vi "BCU诊断标定.vi"(8 "CAN端口":u16(ring), 9 "设备索引号":u16(ring), 10 "CAN卡类型":u32(ring)=21, 11 "Myindex":dbl=1.0) -> (3 "成功":bool)   [LabVIEW 2013] (continued)
            n1896 = event-data() -> ("NewVal"=w2288:bool)  [unwired: 6 out]
            n1897 = case shown="真" w2288 {
              tunnel: w2292 -> [w2294 w2300]
              tunnel: [w2294 w2299] -> w2291
              tunnel: w2290 -> [w2293 w2298]
              tunnel: [w2293 w2297] -> w2289
              frame False {
              }
              frame True {
                n1898 = local write "布尔"(TRUE ("布尔")) -> ()
                n1899 = Enqueue Element(queue=w2300, element="读配置文件", error in (no error)=w2298) -> (queue out=w2299:refnum<queue>, error out=w2297:errorcluster)  [unwired: 2 out]
                n1900 = call <vilib>:"Set Busy.vi"() -> ()  [unwired: 4 in, 8 out]
              }
            }
          }
          event "保存主板参数": Value Change {
            n1901 = event-data() -> ("NewVal"=w2301:bool)  [unwired: 6 out]
            n1902 = case shown="真" w2301 {
              tunnel: w2305 -> [w2307 w2312]
              tunnel: [w2307 w2311] -> w2304
              tunnel: w2303 -> [w2306 w2310]
              tunnel: [w2306 w2309] -> w2302
              frame False {
              }
              frame True {
                n1903 = call <vilib>:"Set Busy.vi"() -> ()  [unwired: 4 in, 8 out]
                n1904 = Enqueue Element(queue=w2312, element="写配置文件", error in (no error)=w2310) -> (queue out=w2311:refnum<queue>, error out=w2309:errorcluster)  [unwired: 2 out]
              }
            }
          }
          event "继电器全开": Value Change {
            n1905 = event-data() -> ("NewVal"=w2313:bool)  [unwired: 6 out]
            n1906 = case shown="真" w2313 {
              tunnel: w2313 -> [_ w2316]
              frame False {
              }
              frame True {
                n1907 = stacked-sequence {
                  tunnel: w2316 -> [_ w2326 _]
                  frame #0 {
                    w2317 = FALSE ("清BUFF")
                    n1908 = local write "正级继电器"(w2317) -> ()
                    n1909 = local write "负级继电器"(w2317) -> ()
                    n1910 = local write "充电继电器"(w2317) -> ()
                    n1911 = local write "加热继电器"(w2317) -> ()
                    n1912 = local write "风机继电器"(w2317) -> ()
                    n1913 = local write "预充电继电器"(w2317) -> ()
                    n1914 = local write "继电器超时处理"(FALSE ("继电器超时处理")) -> ()
                    n1915 = local write "主从选择"(enum32{"主板", "从板"}."主板" ("主从选择")) -> ()
                    n1916 = local write "清BUFF"(FALSE ("清BUFF")) -> ()
                  }
                  frame #1 {
                    n1917 = case shown="真" w2326 {
                      selector: w2326 -> [_ w2341]
                      frame False {
                      }
                      frame True {
                        w2337 = 256.0 ("y")
                        w2328 = u32 1 ("命令序号")
                        w2327 = u8 192 ("命令")
                        n1918 = local read "动作保持时间"() -> (w2338:dbl)
                        n1919 = Quotient & Remainder(x=w2338, y=w2337) -> (x-y*floor(x/y)=w2330:dbl, floor(x/y)=w2334:dbl)
                        n1920 = Quotient & Remainder(x=w2334, y=w2337) -> (x-y*floor(x/y)=w2331:dbl, floor(x/y)=w2335:dbl)
                        n1921 = Quotient & Remainder(x=w2335, y=w2337) -> (x-y*floor(x/y)=w2332:dbl, floor(x/y)=w2336:dbl)
                        n1922 = local read "设备索引号"() -> (w2345:u16)
                        n1923 = local read "CAN卡类型"() -> (w2346:u32)
                        n1924 = local read "CAN端口"() -> (w2344:u16)
                        n1925 = Boolean To (0,1)(Boolean=w2341) -> (0, 1=w2339:i16)
                        n1926 = Quotient & Remainder(x=w2336, y=w2337) -> (x-y*floor(x/y)=w2333:dbl)  [unwired: 1 out]
                        n1927 = Build Array(i16 170 ("元素"), w2339, w2333, w2332, w2331, w2330, 0.0 ("元素")) -> (w2342:dbl[])
                        n1928 = call "多帧发送机制(EV05).vi"("can卡类型"=w2346, "设备索引号"=w2345, "CAN端口"=w2344, "命令"=w2327, "板号"=u8 0, "命令序号"=w2328, "输入数据"=w2342) -> ()  [unwired: 2 in, 11 out]
                        n1929 = local write "命令序号"(w2328) -> ()
                        n1930 = local write "命令"(w2327) -> ()
                      }
                    }
                    n1931 = local write "控制1"(TRUE ("控制1")) -> ()
                    n1932 = local write "写?"(FALSE ("写?")) -> ()
                    n1933 = local write "消除"(TRUE ("消除")) -> ()
                    n1934 = global write "EV05全局变量1.vi" "流控帧 2"(TRUE ("流控帧 2")) -> ()
                    n1935 = global write "EV05全局变量1.vi" "流控帧"(FALSE ("流控帧")) -> ()
                  }
                  frame #2 {
                    n1936 = flat-sequence {
                      tunnel: [w2348] -> w2347
                      tunnel: w2347 -> [w2355]
                      frame #0 {
                        n1937 = while {
                          tunnel: [w2349] -> w2348
                          i -> [w2353]
                          stop <- w2350 stop-if-true
                          n1938 = local read "继电器超时处理"() -> (w2349:bool)
                          n1939 = Greater Or Equal?(x=w2353, y=20) -> (x >= y?=w2351:bool)
                          n1940 = Wait Until Next ms Multiple(millisecond multiple=u32 100 ("毫秒倍数")) -> ()  [unwired: 1 out]
                          n1941 = Or(x=w2349, y=w2351) -> (x .or. y?=w2350:bool)
                        }
                      }
                      frame #1 {
                        n1942 = case shown="真" w2355 {
                          frame False {
                            n1943 = One Button Dialog(message="继电器处理超时" ("消息"), button name ("OK")="是" ("按钮名称（“确定”）")) -> ()  [unwired: 1 out]
                          }
                          frame True {
                            w2358 = TRUE ("清BUFF")
                            n1944 = local write "正级继电器"(w2358) -> ()
                            n1945 = local write "负级继电器"(w2358) -> ()
                            n1946 = local write "充电继电器"(w2358) -> ()
                            n1947 = local write "加热继电器"(w2358) -> ()
                            n1948 = local write "风机继电器"(w2358) -> ()
                            n1949 = local write "预充电继电器"(w2358) -> ()
                          }
                        }
                      }
                    }
                  }
                }
              }
            }
          }
          event "继电器全关": Value Change {
            n1950 = event-data() -> ("NewVal"=w2359:bool)  [unwired: 6 out]
            n1951 = case shown="真" w2359 {
              tunnel: w2359 -> [_ w2362]
              frame False {
              }
              frame True {
                n1952 = stacked-sequence {
                  tunnel: w2362 -> [_ w2372 _]
                  frame #0 {
                    w2363 = TRUE ("清BUFF")
                    n1953 = local write "正级继电器"(w2363) -> ()
                    n1954 = local write "负级继电器"(w2363) -> ()
                    n1955 = local write "充电继电器"(w2363) -> ()
                    n1956 = local write "加热继电器"(w2363) -> ()
                    n1957 = local write "风机继电器"(w2363) -> ()
                    n1958 = local write "预充电继电器"(w2363) -> ()
                    n1959 = local write "继电器超时处理"(FALSE ("继电器超时处理")) -> ()
                    n1960 = local write "主从选择"(enum32{"主板", "从板"}."主板" ("主从选择")) -> ()
                    n1961 = global write "EV05全局变量1.vi" "流控帧"(FALSE ("流控帧")) -> ()
                    n1962 = local write "清BUFF"(FALSE ("清BUFF")) -> ()
                  }
                  frame #1 {
                    n1963 = case shown="真" w2372 {
                      selector: w2372 -> [_ w2387]
                      frame False {
                      }
                      frame True {
                        w2383 = 256.0 ("y")
                        w2374 = u32 1 ("命令序号")
                        w2373 = u8 192 ("命令")
                        n1964 = local read "动作保持时间"() -> (w2384:dbl)
                        n1965 = Quotient & Remainder(x=w2384, y=w2383) -> (x-y*floor(x/y)=w2376:dbl, floor(x/y)=w2380:dbl)
                        n1966 = Quotient & Remainder(x=w2380, y=w2383) -> (x-y*floor(x/y)=w2377:dbl, floor(x/y)=w2381:dbl)
                        n1967 = Quotient & Remainder(x=w2381, y=w2383) -> (x-y*floor(x/y)=w2378:dbl, floor(x/y)=w2382:dbl)
                        n1968 = local read "设备索引号"() -> (w2391:u16)
                        n1969 = local read "CAN卡类型"() -> (w2392:u32)
                        n1970 = local read "CAN端口"() -> (w2390:u16)
                        n1971 = Boolean To (0,1)(Boolean=w2387) -> (0, 1=w2385:i16)
                        n1972 = Quotient & Remainder(x=w2382, y=w2383) -> (x-y*floor(x/y)=w2379:dbl)  [unwired: 1 out]
                        n1973 = Build Array(i16 85 ("元素"), w2385, w2379, w2378, w2377, w2376, 0.0 ("元素")) -> (w2388:dbl[])
                        n1974 = call "多帧发送机制(EV05).vi"("can卡类型"=w2392, "设备索引号"=w2391, "CAN端口"=w2390, "命令"=w2373, "板号"=u8 0, "命令序号"=w2374, "输入数据"=w2388) -> ()  [unwired: 2 in, 11 out]
                        n1975 = local write "命令序号"(w2374) -> ()
                        n1976 = local write "命令"(w2373) -> ()
                      }
                    }
                    n1977 = local write "控制1"(TRUE ("控制1")) -> ()
                    n1978 = local write "写?"(FALSE ("写?")) -> ()
                    n1979 = local write "消除"(TRUE ("消除")) -> ()
                    n1980 = global write "EV05全局变量1.vi" "流控帧 2"(TRUE ("流控帧 2")) -> ()
                  }
                  frame #2 {
                    n1981 = flat-sequence {
                      tunnel: [w2394] -> w2393
                      tunnel: w2393 -> [w2401]
                      frame #0 {
                        n1982 = while {
                          tunnel: [w2395] -> w2394
                          i -> [w2399]
                          stop <- w2396 stop-if-true
                          n1983 = local read "继电器超时处理"() -> (w2395:bool)
                          n1984 = Greater Or Equal?(x=w2399, y=20) -> (x >= y?=w2397:bool)
                          n1985 = Wait Until Next ms Multiple(millisecond multiple=u32 100 ("毫秒倍数")) -> ()  [unwired: 1 out]
                          n1986 = Or(x=w2395, y=w2397) -> (x .or. y?=w2396:bool)
                        }
                      }
                      frame #1 {
                        n1987 = case shown="真" w2401 {
                          frame False {
                            n1988 = One Button Dialog(message="继电器处理超时" ("消息"), button name ("OK")="是" ("按钮名称（“确定”）")) -> ()  [unwired: 1 out]
                          }
                          frame True {
                            w2404 = FALSE ("清BUFF")
                            n1989 = local write "正级继电器"(w2404) -> ()
                            n1990 = local write "负级继电器"(w2404) -> ()
                            n1991 = local write "充电继电器"(w2404) -> ()
                            n1992 = local write "加热继电器"(w2404) -> ()
                            n1993 = local write "风机继电器"(w2404) -> ()
                            n1994 = local write "预充电继电器"(w2404) -> ()
                          }
                        }
                      }
                    }
                  }
                }
              }
            }
          }
          event "控制按键全为开": Value Change {
            n1995 = event-data() -> ("NewVal"=w2405:bool)  [unwired: 6 out]
            n1996 = case shown="真" w2405 {
              frame False {
              }
              frame True {
                w2406 = TRUE ("正级继电器")
                n1997 = local write "加热继电器(从)"(w2406) -> ()
                n1998 = local write "风机继电器(从)"(w2406) -> ()
                n1999 = local write "DO1 2"(w2406) -> ()
                n2000 = local write "DO1"(w2406) -> ()
                n2001 = local write "DO2"(w2406) -> ()
                n2002 = local write "正级继电器"(w2406) -> ()
                n2003 = local write "负级继电器"(w2406) -> ()
                n2004 = local write "加热继电器"(w2406) -> ()
                n2005 = local write "预充电继电器"(w2406) -> ()
                n2006 = local write "充电继电器"(w2406) -> ()
                n2007 = local write "风机继电器"(w2406) -> ()
              }
            }
          }
          event "控制按键全为关": Value Change {
            n2008 = event-data() -> ("NewVal"=w2407:bool)  [unwired: 6 out]
            n2009 = case shown="真" w2407 {
              frame False {
              }
              frame True {
                w2408 = FALSE ("正级继电器")
                n2010 = local write "加热继电器(从)"(w2408) -> ()
                n2011 = local write "风机继电器(从)"(w2408) -> ()
                n2012 = local write "DO1 2"(w2408) -> ()
                n2013 = local write "DO1"(w2408) -> ()
                n2014 = local write "DO2"(w2408) -> ()
                n2015 = local write "正级继电器"(w2408) -> ()
                n2016 = local write "负级继电器"(w2408) -> ()
                n2017 = local write "加热继电器"(w2408) -> ()
                n2018 = local write "预充电继电器"(w2408) -> ()
                n2019 = local write "充电继电器"(w2408) -> ()
                n2020 = local write "风机继电器"(w2408) -> ()
              }
            }
          }
          event "正级继电器": Value Change {
            n2021 = event-data() -> ("NewVal"=w2409:bool)  [unwired: 6 out]
            n2022 = stacked-sequence {
              tunnel: w2409 -> [_ w2422 _]
              frame #0 {
                w2412 = FALSE ("清BUFF")
                n2023 = local write "继电器超时处理"(FALSE ("继电器超时处理")) -> ()
                n2024 = local write "主从选择"(enum32{"主板", "从板"}."主板" ("主从选择")) -> ()
                n2025 = local write "正级继电器 12"(w2412) -> ()
                n2026 = local write "清BUFF"(w2412) -> ()
              }
              frame #1 {
                n2027 = case shown="假" w2422 {
                  selector: w2422 -> [w2437 w2457]
                  tunnel: [w2436 w2456] -> w2421
                  tunnel: [w2424 w2444] -> w2416
                  frame False {
                    w2432 = 256.0 ("y")
                    w2424 = u32 1 ("命令序号")
                    w2436 = u8 192 ("命令")
                    n2028 = local read "动作保持时间"() -> (w2433:dbl)
                    n2029 = Quotient & Remainder(x=w2433, y=w2432) -> (x-y*floor(x/y)=w2425:dbl, floor(x/y)=w2429:dbl)
                    n2030 = Quotient & Remainder(x=w2429, y=w2432) -> (x-y*floor(x/y)=w2426:dbl, floor(x/y)=w2430:dbl)
                    n2031 = Quotient & Remainder(x=w2430, y=w2432) -> (x-y*floor(x/y)=w2427:dbl, floor(x/y)=w2431:dbl)
                    n2032 = local read "设备索引号"() -> (w2441:u16)
                    n2033 = local read "CAN卡类型"() -> (w2442:u32)
                    n2034 = local read "CAN端口"() -> (w2440:u16)
                    n2035 = Boolean To (0,1)(Boolean=w2437) -> (0, 1=w2434:i16)
                    n2036 = Quotient & Remainder(x=w2431, y=w2432) -> (x-y*floor(x/y)=w2428:dbl)  [unwired: 1 out]
                    n2037 = Build Array(i16 1 ("元素"), w2434, w2428, w2427, w2426, w2425, 0.0 ("元素")) -> (w2438:dbl[])
                    n2038 = call "多帧发送机制(EV05).vi"("can卡类型"=w2442, "设备索引号"=w2441, "CAN端口"=w2440, "命令"=w2436, "板号"=u8 0, "命令序号"=w2424, "输入数据"=w2438) -> ()  [unwired: 2 in, 11 out]
                  }
                  frame True {
                    w2452 = 256.0 ("y")
                    w2444 = u32 1 ("命令序号")
                    w2456 = u8 192 ("命令")
                    n2039 = local read "动作保持时间"() -> (w2453:dbl)
                    n2040 = Quotient & Remainder(x=w2453, y=w2452) -> (x-y*floor(x/y)=w2445:dbl, floor(x/y)=w2449:dbl)
                    n2041 = Quotient & Remainder(x=w2449, y=w2452) -> (x-y*floor(x/y)=w2446:dbl, floor(x/y)=w2450:dbl)
                    n2042 = Quotient & Remainder(x=w2450, y=w2452) -> (x-y*floor(x/y)=w2447:dbl, floor(x/y)=w2451:dbl)
                    n2043 = local read "设备索引号"() -> (w2461:u16)
                    n2044 = local read "CAN卡类型"() -> (w2462:u32)
                    n2045 = local read "CAN端口"() -> (w2460:u16)
                    n2046 = Boolean To (0,1)(Boolean=w2457) -> (0, 1=w2454:i16)
                    n2047 = Quotient & Remainder(x=w2451, y=w2452) -> (x-y*floor(x/y)=w2448:dbl)  [unwired: 1 out]
                    n2048 = Build Array(i16 1 ("元素"), w2454, w2448, w2447, w2446, w2445, 0.0 ("元素")) -> (w2458:dbl[])
                    n2049 = call "多帧发送机制(EV05).vi"("can卡类型"=w2462, "设备索引号"=w2461, "CAN端口"=w2460, "命令"=w2456, "板号"=u8 0, "命令序号"=w2444, "输入数据"=w2458) -> ()  [unwired: 2 in, 11 out]
                  }
                }
                n2050 = local write "命令序号"(w2416) -> ()
                n2051 = local write "命令"(w2421) -> ()
                n2052 = local write "控制1"(TRUE ("控制1")) -> ()
                n2053 = local write "写?"(FALSE ("写?")) -> ()
                n2054 = global write "EV05全局变量1.vi" "流控帧"(FALSE ("流控帧")) -> ()
                n2055 = local write "消除"(TRUE ("消除")) -> ()
                n2056 = global write "EV05全局变量1.vi" "流控帧 2"(TRUE ("流控帧 2")) -> ()
              }
              frame #2 {
                n2057 = flat-sequence {
                  tunnel: [w2464] -> w2463
                  tunnel: w2463 -> [w2471]
                  frame #0 {
                    n2058 = while {
                      tunnel: [w2465] -> w2464
                      i -> [w2469]
                      stop <- w2466 stop-if-true
                      n2059 = local read "继电器超时处理"() -> (w2465:bool)
                      n2060 = Greater Or Equal?(x=w2469, y=20) -> (x >= y?=w2467:bool)
                      n2061 = Wait Until Next ms Multiple(millisecond multiple=u32 100 ("毫秒倍数")) -> ()  [unwired: 1 out]
                      n2062 = Or(x=w2465, y=w2467) -> (x .or. y?=w2466:bool)
                    }
                  }
                  frame #1 {
                    n2063 = case shown="假" w2471 {
                      frame False {
                        n2064 = local read "正级继电器"() -> (w2473:bool)
                        n2065 = Not(x=w2473) -> (.not. x?=w2472:bool)
                        n2066 = local write "正级继电器"(w2472) -> ()
                        n2067 = One Button Dialog(message="继电器处理超时" ("消息"), button name ("OK")="是" ("按钮名称（“确定”）")) -> ()  [unwired: 1 out]
                      }
                      frame True {
                      }
                    }
                  }
                }
              }
            }
          }
          event "负级继电器": Value Change {
            n2068 = event-data() -> ("NewVal"=w2476:bool)  [unwired: 6 out]
            n2069 = stacked-sequence {
              tunnel: w2476 -> [_ w2489 _]
              frame #0 {
                w2479 = FALSE ("继电器超时处理")
                n2070 = local write "继电器超时处理"(w2479) -> ()
                n2071 = local write "正级继电器 2"(w2479) -> ()
                n2072 = local write "主从选择"(enum32{"主板", "从板"}."主板" ("主从选择")) -> ()
              }
              frame #1 {
                n2073 = case shown="假" w2489 {
                  selector: w2489 -> [w2503 w2523]
                  tunnel: [w2502 w2522] -> w2488
                  tunnel: [w2491 w2511] -> w2483
                  frame False {
                    w2499 = 256.0 ("y")
                    w2491 = u32 1 ("命令序号")
                    w2502 = u8 192 ("命令")
                    n2074 = local read "动作保持时间"() -> (w2500:dbl)
                    n2075 = Quotient & Remainder(x=w2500, y=w2499) -> (x-y*floor(x/y)=w2492:dbl, floor(x/y)=w2496:dbl)
                    n2076 = Quotient & Remainder(x=w2496, y=w2499) -> (x-y*floor(x/y)=w2493:dbl, floor(x/y)=w2497:dbl)
                    n2077 = Quotient & Remainder(x=w2497, y=w2499) -> (x-y*floor(x/y)=w2494:dbl, floor(x/y)=w2498:dbl)
                    n2078 = Quotient & Remainder(x=w2498, y=w2499) -> (x-y*floor(x/y)=w2495:dbl)  [unwired: 1 out]
                    n2079 = Boolean To (0,1)(Boolean=w2503) -> (0, 1=w2501:i16)
                    n2080 = local read "设备索引号"() -> (w2508:u16)
                    n2081 = local read "CAN卡类型"() -> (w2509:u32)
                    n2082 = local read "CAN端口"() -> (w2507:u16)
                    n2083 = Build Array(i16 2 ("元素"), w2501, w2495, w2494, w2493, w2492, 0.0 ("元素")) -> (w2505:dbl[])
                    n2084 = call "多帧发送机制(EV05).vi"("can卡类型"=w2509, "设备索引号"=w2508, "CAN端口"=w2507, "命令"=w2502, "板号"=u8 0, "命令序号"=w2491, "输入数据"=w2505) -> ()  [unwired: 2 in, 11 out]
                  }
                  frame True {
                    w2519 = 256.0 ("y")
                    w2511 = u32 1 ("命令序号")
                    w2522 = u8 192 ("命令")
                    n2085 = local read "动作保持时间"() -> (w2520:dbl)
                    n2086 = Quotient & Remainder(x=w2520, y=w2519) -> (x-y*floor(x/y)=w2512:dbl, floor(x/y)=w2516:dbl)
                    n2087 = Quotient & Remainder(x=w2516, y=w2519) -> (x-y*floor(x/y)=w2513:dbl, floor(x/y)=w2517:dbl)
                    n2088 = Quotient & Remainder(x=w2517, y=w2519) -> (x-y*floor(x/y)=w2514:dbl, floor(x/y)=w2518:dbl)
                    n2089 = Quotient & Remainder(x=w2518, y=w2519) -> (x-y*floor(x/y)=w2515:dbl)  [unwired: 1 out]
                    n2090 = Boolean To (0,1)(Boolean=w2523) -> (0, 1=w2521:i16)
                    n2091 = local read "设备索引号"() -> (w2528:u16)
                    n2092 = local read "CAN卡类型"() -> (w2529:u32)
                    n2093 = local read "CAN端口"() -> (w2527:u16)
                    n2094 = Build Array(i16 2 ("元素"), w2521, w2515, w2514, w2513, w2512, 0.0 ("元素")) -> (w2525:dbl[])
                    n2095 = call "多帧发送机制(EV05).vi"("can卡类型"=w2529, "设备索引号"=w2528, "CAN端口"=w2527, "命令"=w2522, "板号"=u8 0, "命令序号"=w2511, "输入数据"=w2525) -> ()  [unwired: 2 in, 11 out]
                  }
                }
                n2096 = local write "命令"(w2488) -> ()
                n2097 = local write "命令序号"(w2483) -> ()
                n2098 = local write "清BUFF"(FALSE ("清BUFF")) -> ()
                n2099 = global write "EV05全局变量1.vi" "流控帧"(FALSE ("流控帧")) -> ()
                n2100 = local write "控制1"(TRUE ("控制1")) -> ()
                n2101 = global write "EV05全局变量1.vi" "流控帧 2"(TRUE ("流控帧 2")) -> ()
                n2102 = local write "写?"(FALSE ("写?")) -> ()
                n2103 = local write "消除"(TRUE ("消除")) -> ()
              }
              frame #2 {
                n2104 = flat-sequence {
                  tunnel: [w2531] -> w2530
                  tunnel: w2530 -> [w2538]
                  frame #0 {
                    n2105 = while {
                      tunnel: [w2532] -> w2531
                      i -> [w2536]
                      stop <- w2533 stop-if-true
                      n2106 = local read "继电器超时处理"() -> (w2532:bool)
                      n2107 = Greater Or Equal?(x=w2536, y=20) -> (x >= y?=w2534:bool)
                      n2108 = Wait Until Next ms Multiple(millisecond multiple=u32 100 ("毫秒倍数")) -> ()  [unwired: 1 out]
                      n2109 = Or(x=w2532, y=w2534) -> (x .or. y?=w2533:bool)
                    }
                  }
                  frame #1 {
                    n2110 = case shown="假" w2538 {
                      frame False {
                        n2111 = local read "负级继电器"() -> (w2539:bool)
                        n2112 = Not(x=w2539) -> (.not. x?=w2540:bool)
                        n2113 = local write "负级继电器"(w2540) -> ()
                        n2114 = One Button Dialog(message="继电器处理超时" ("消息"), button name ("OK")="是" ("按钮名称（“确定”）")) -> ()  [unwired: 1 out]
                      }
                      frame True {
                      }
                    }
                  }
                }
              }
            }
          }
          event "预充电继电器": Value Change {
            n2115 = event-data() -> ("NewVal"=w2543:bool)  [unwired: 6 out]
            n2116 = stacked-sequence {
              tunnel: w2543 -> [_ w2556 _]
              frame #0 {
                w2547 = FALSE ("继电器超时处理")
                n2117 = local write "继电器超时处理"(w2547) -> ()
                n2118 = local write "正级继电器 3"(w2547) -> ()
                n2119 = global write "EV05全局变量1.vi" "流控帧"(FALSE ("流控帧")) -> ()
                n2120 = local write "主从选择"(enum32{"主板", "从板"}."主板" ("主从选择")) -> ()
              }
              frame #1 {
                n2121 = case shown="假" w2556 {
                  selector: w2556 -> [w2570 w2590]
                  tunnel: [w2569 w2589] -> w2555
                  tunnel: [w2558 w2578] -> w2550
                  frame False {
                    w2566 = 256.0 ("y")
                    w2558 = u32 1 ("命令序号")
                    w2569 = u8 192 ("命令")
                    n2122 = local read "动作保持时间"() -> (w2567:dbl)
                    n2123 = Quotient & Remainder(x=w2567, y=w2566) -> (x-y*floor(x/y)=w2559:dbl, floor(x/y)=w2563:dbl)
                    n2124 = Quotient & Remainder(x=w2563, y=w2566) -> (x-y*floor(x/y)=w2560:dbl, floor(x/y)=w2564:dbl)
                    n2125 = Quotient & Remainder(x=w2564, y=w2566) -> (x-y*floor(x/y)=w2561:dbl, floor(x/y)=w2565:dbl)
                    n2126 = Quotient & Remainder(x=w2565, y=w2566) -> (x-y*floor(x/y)=w2562:dbl)  [unwired: 1 out]
                    n2127 = Boolean To (0,1)(Boolean=w2570) -> (0, 1=w2568:i16)
                    n2128 = local read "设备索引号"() -> (w2575:u16)
                    n2129 = local read "CAN卡类型"() -> (w2576:u32)
                    n2130 = local read "CAN端口"() -> (w2574:u16)
                    n2131 = Build Array(i16 3 ("元素"), w2568, w2562, w2561, w2560, w2559, 0.0 ("元素")) -> (w2572:dbl[])
                    n2132 = call "多帧发送机制(EV05).vi"("can卡类型"=w2576, "设备索引号"=w2575, "CAN端口"=w2574, "命令"=w2569, "板号"=u8 0, "命令序号"=w2558, "输入数据"=w2572) -> ()  [unwired: 2 in, 11 out]
                  }
                  frame True {
                    w2586 = 256.0 ("y")
                    w2578 = u32 1 ("命令序号")
                    w2589 = u8 192 ("命令")
                    n2133 = local read "动作保持时间"() -> (w2587:dbl)
                    n2134 = Quotient & Remainder(x=w2587, y=w2586) -> (x-y*floor(x/y)=w2579:dbl, floor(x/y)=w2583:dbl)
                    n2135 = Quotient & Remainder(x=w2583, y=w2586) -> (x-y*floor(x/y)=w2580:dbl, floor(x/y)=w2584:dbl)
                    n2136 = Quotient & Remainder(x=w2584, y=w2586) -> (x-y*floor(x/y)=w2581:dbl, floor(x/y)=w2585:dbl)
                    n2137 = Quotient & Remainder(x=w2585, y=w2586) -> (x-y*floor(x/y)=w2582:dbl)  [unwired: 1 out]
                    n2138 = Boolean To (0,1)(Boolean=w2590) -> (0, 1=w2588:i16)
                    n2139 = local read "设备索引号"() -> (w2595:u16)
                    n2140 = local read "CAN卡类型"() -> (w2596:u32)
                    n2141 = local read "CAN端口"() -> (w2594:u16)
                    n2142 = Build Array(i16 3 ("元素"), w2588, w2582, w2581, w2580, w2579, 0.0 ("元素")) -> (w2592:dbl[])
                    n2143 = call "多帧发送机制(EV05).vi"("can卡类型"=w2596, "设备索引号"=w2595, "CAN端口"=w2594, "命令"=w2589, "板号"=u8 0, "命令序号"=w2578, "输入数据"=w2592) -> ()  [unwired: 2 in, 11 out]
                  }
                }
                n2144 = local write "命令序号"(w2550) -> ()
                n2145 = local write "清BUFF"(FALSE ("清BUFF")) -> ()
                n2146 = local write "控制1"(TRUE ("控制1")) -> ()
                n2147 = global write "EV05全局变量1.vi" "流控帧 2"(TRUE ("流控帧 2")) -> ()
                n2148 = local write "消除"(TRUE ("消除")) -> ()
                n2149 = local write "命令"(w2555) -> ()
                n2150 = local write "写?"(FALSE ("写?")) -> ()
              }
              frame #2 {
                n2151 = flat-sequence {
                  tunnel: [w2598] -> w2597
                  tunnel: w2597 -> [w2605]
                  frame #0 {
                    n2152 = while {
                      tunnel: [w2599] -> w2598
                      i -> [w2603]
                      stop <- w2600 stop-if-true
                      n2153 = local read "继电器超时处理"() -> (w2599:bool)
                      n2154 = Greater Or Equal?(x=w2603, y=20) -> (x >= y?=w2601:bool)
                      n2155 = Wait Until Next ms Multiple(millisecond multiple=u32 100 ("毫秒倍数")) -> ()  [unwired: 1 out]
                      n2156 = Or(x=w2599, y=w2601) -> (x .or. y?=w2600:bool)
                    }
                  }
                  frame #1 {
                    n2157 = case shown="假" w2605 {
                      frame False {
                        n2158 = local read "预充电继电器"() -> (w2606:bool)
                        n2159 = Not(x=w2606) -> (.not. x?=w2607:bool)
                        n2160 = local write "预充电继电器"(w2607) -> ()
                        n2161 = One Button Dialog(message="继电器处理超时" ("消息"), button name ("OK")="是" ("按钮名称（“确定”）")) -> ()  [unwired: 1 out]
                      }
                      frame True {
                      }
                    }
                  }
                }
              }
            }
          }
          event "加热继电器": Value Change {
            n2162 = event-data() -> ("NewVal"=w2610:bool)  [unwired: 6 out]
            n2163 = stacked-sequence {
              tunnel: w2610 -> [_ w2623 _]
              frame #0 {
                w2614 = FALSE ("继电器超时处理")
                n2164 = local write "继电器超时处理"(w2614) -> ()
                n2165 = local write "正级继电器 5"(w2614) -> ()
                n2166 = global write "EV05全局变量1.vi" "流控帧"(FALSE ("流控帧")) -> ()
                n2167 = local write "主从选择"(enum32{"主板", "从板"}."主板" ("主从选择")) -> ()
              }
              frame #1 {
                n2168 = case shown="假" w2623 {
                  selector: w2623 -> [w2637 w2657]
                  tunnel: [w2636 w2656] -> w2622
                  tunnel: [w2625 w2645] -> w2617
                  frame False {
                    w2633 = 256.0 ("y")
                    w2625 = u32 1 ("命令序号")
                    w2636 = u8 192 ("命令")
                    n2169 = local read "动作保持时间"() -> (w2634:dbl)
                    n2170 = Quotient & Remainder(x=w2634, y=w2633) -> (x-y*floor(x/y)=w2626:dbl, floor(x/y)=w2630:dbl)
                    n2171 = Quotient & Remainder(x=w2630, y=w2633) -> (x-y*floor(x/y)=w2627:dbl, floor(x/y)=w2631:dbl)
                    n2172 = Quotient & Remainder(x=w2631, y=w2633) -> (x-y*floor(x/y)=w2628:dbl, floor(x/y)=w2632:dbl)
                    n2173 = Quotient & Remainder(x=w2632, y=w2633) -> (x-y*floor(x/y)=w2629:dbl)  [unwired: 1 out]
                    n2174 = Boolean To (0,1)(Boolean=w2637) -> (0, 1=w2635:i16)
                    n2175 = local read "设备索引号"() -> (w2642:u16)
                    n2176 = local read "CAN卡类型"() -> (w2643:u32)
                    n2177 = local read "CAN端口"() -> (w2641:u16)
                    n2178 = Build Array(i16 4 ("元素"), w2635, w2629, w2628, w2627, w2626, 0.0 ("元素")) -> (w2639:dbl[])
                    n2179 = call "多帧发送机制(EV05).vi"("can卡类型"=w2643, "设备索引号"=w2642, "CAN端口"=w2641, "命令"=w2636, "板号"=u8 0, "命令序号"=w2625, "输入数据"=w2639) -> ()  [unwired: 2 in, 11 out]
                  }
                  frame True {
                    w2653 = 256.0 ("y")
                    w2645 = u32 1 ("命令序号")
                    w2656 = u8 192 ("命令")
                    n2180 = local read "动作保持时间"() -> (w2654:dbl)
                    n2181 = Quotient & Remainder(x=w2654, y=w2653) -> (x-y*floor(x/y)=w2646:dbl, floor(x/y)=w2650:dbl)
                    n2182 = Quotient & Remainder(x=w2650, y=w2653) -> (x-y*floor(x/y)=w2647:dbl, floor(x/y)=w2651:dbl)
                    n2183 = Quotient & Remainder(x=w2651, y=w2653) -> (x-y*floor(x/y)=w2648:dbl, floor(x/y)=w2652:dbl)
                    n2184 = Quotient & Remainder(x=w2652, y=w2653) -> (x-y*floor(x/y)=w2649:dbl)  [unwired: 1 out]
                    n2185 = Boolean To (0,1)(Boolean=w2657) -> (0, 1=w2655:i16)
                    n2186 = local read "设备索引号"() -> (w2662:u16)
                    n2187 = local read "CAN卡类型"() -> (w2663:u32)
                    n2188 = local read "CAN端口"() -> (w2661:u16)
                    n2189 = Build Array(i16 4 ("元素"), w2655, w2649, w2648, w2647, w2646, 0.0 ("元素")) -> (w2659:dbl[])
                    n2190 = call "多帧发送机制(EV05).vi"("can卡类型"=w2663, "设备索引号"=w2662, "CAN端口"=w2661, "命令"=w2656, "板号"=u8 0, "命令序号"=w2645, "输入数据"=w2659) -> ()  [unwired: 2 in, 11 out]
                  }
                }
                n2191 = local write "命令序号"(w2617) -> ()
                n2192 = local write "清BUFF"(FALSE ("清BUFF")) -> ()
                n2193 = local write "命令"(w2622) -> ()
                n2194 = local write "控制1"(TRUE ("控制1")) -> ()
                n2195 = local write "写?"(FALSE ("写?")) -> ()
                n2196 = global write "EV05全局变量1.vi" "流控帧 2"(TRUE ("流控帧 2")) -> ()
                n2197 = local write "消除"(TRUE ("消除")) -> ()
              }
              frame #2 {
                n2198 = flat-sequence {
                  tunnel: [w2665] -> w2664
                  tunnel: w2664 -> [w2672]
                  frame #0 {
                    n2199 = while {
                      tunnel: [w2666] -> w2665
                      i -> [w2670]
                      stop <- w2667 stop-if-true
                      n2200 = local read "继电器超时处理"() -> (w2666:bool)
                      n2201 = Greater Or Equal?(x=w2670, y=20) -> (x >= y?=w2668:bool)
                      n2202 = Wait Until Next ms Multiple(millisecond multiple=u32 100 ("毫秒倍数")) -> ()  [unwired: 1 out]
                      n2203 = Or(x=w2666, y=w2668) -> (x .or. y?=w2667:bool)
                    }
                  }
                  frame #1 {
                    n2204 = case shown="假" w2672 {
                      frame False {
                        n2205 = local read "加热继电器"() -> (w2673:bool)
                        n2206 = Not(x=w2673) -> (.not. x?=w2674:bool)
                        n2207 = local write "加热继电器"(w2674) -> ()
                        n2208 = One Button Dialog(message="继电器处理超时" ("消息"), button name ("OK")="是" ("按钮名称（“确定”）")) -> ()  [unwired: 1 out]
                      }
                      frame True {
                      }
                    }
                  }
                }
              }
            }
          }
          event "充电继电器": Value Change {
            n2209 = event-data() -> ("NewVal"=w2677:bool)  [unwired: 6 out]
            n2210 = stacked-sequence {
              tunnel: w2677 -> [_ w2690 _]
              frame #0 {
                w2681 = FALSE ("继电器超时处理")
                n2211 = local write "主从选择"(enum32{"主板", "从板"}."主板" ("主从选择")) -> ()
                n2212 = global write "EV05全局变量1.vi" "流控帧"(FALSE ("流控帧")) -> ()
                n2213 = local write "继电器超时处理"(w2681) -> ()
                n2214 = local write "正级继电器 4"(w2681) -> ()
              }
              frame #1 {
                n2215 = case shown="假" w2690 {
                  selector: w2690 -> [w2704 w2724]
                  tunnel: [w2703 w2723] -> w2689
                  tunnel: [w2692 w2712] -> w2684
                  frame False {
                    w2700 = 256.0 ("y")
                    w2692 = u32 1 ("命令序号")
                    w2703 = u8 192 ("命令")
                    n2216 = local read "动作保持时间"() -> (w2701:dbl)
                    n2217 = Quotient & Remainder(x=w2701, y=w2700) -> (x-y*floor(x/y)=w2693:dbl, floor(x/y)=w2697:dbl)
                    n2218 = Quotient & Remainder(x=w2697, y=w2700) -> (x-y*floor(x/y)=w2694:dbl, floor(x/y)=w2698:dbl)
                    n2219 = Quotient & Remainder(x=w2698, y=w2700) -> (x-y*floor(x/y)=w2695:dbl, floor(x/y)=w2699:dbl)
                    n2220 = Quotient & Remainder(x=w2699, y=w2700) -> (x-y*floor(x/y)=w2696:dbl)  [unwired: 1 out]
                    n2221 = Boolean To (0,1)(Boolean=w2704) -> (0, 1=w2702:i16)
                    n2222 = local read "设备索引号"() -> (w2709:u16)
                    n2223 = local read "CAN卡类型"() -> (w2710:u32)
                    n2224 = local read "CAN端口"() -> (w2708:u16)
                    n2225 = Build Array(i16 5 ("元素"), w2702, w2696, w2695, w2694, w2693, 0.0 ("元素")) -> (w2706:dbl[])
                    n2226 = call "多帧发送机制(EV05).vi"("can卡类型"=w2710, "设备索引号"=w2709, "CAN端口"=w2708, "命令"=w2703, "板号"=u8 0, "命令序号"=w2692, "输入数据"=w2706) -> ()  [unwired: 2 in, 11 out]
                  }
                  frame True {
                    w2720 = 256.0 ("y")
                    w2712 = u32 1 ("命令序号")
                    w2723 = u8 192 ("命令")
                    n2227 = local read "动作保持时间"() -> (w2721:dbl)
                    n2228 = Quotient & Remainder(x=w2721, y=w2720) -> (x-y*floor(x/y)=w2713:dbl, floor(x/y)=w2717:dbl)
                    n2229 = Quotient & Remainder(x=w2717, y=w2720) -> (x-y*floor(x/y)=w2714:dbl, floor(x/y)=w2718:dbl)
                    n2230 = Quotient & Remainder(x=w2718, y=w2720) -> (x-y*floor(x/y)=w2715:dbl, floor(x/y)=w2719:dbl)
                    n2231 = Quotient & Remainder(x=w2719, y=w2720) -> (x-y*floor(x/y)=w2716:dbl)  [unwired: 1 out]
                    n2232 = Boolean To (0,1)(Boolean=w2724) -> (0, 1=w2722:i16)
                    n2233 = local read "设备索引号"() -> (w2729:u16)
                    n2234 = local read "CAN卡类型"() -> (w2730:u32)
                    n2235 = local read "CAN端口"() -> (w2728:u16)
                    n2236 = Build Array(i16 5 ("元素"), w2722, w2716, w2715, w2714, w2713, 0.0 ("元素")) -> (w2726:dbl[])
                    n2237 = call "多帧发送机制(EV05).vi"("can卡类型"=w2730, "设备索引号"=w2729, "CAN端口"=w2728, "命令"=w2723, "板号"=u8 0, "命令序号"=w2712, "输入数据"=w2726) -> ()  [unwired: 2 in, 11 out]
                  }
                }
                n2238 = local write "命令序号"(w2684) -> ()
                n2239 = local write "命令"(w2689) -> ()
                n2240 = local write "清BUFF"(FALSE ("清BUFF")) -> ()
                n2241 = local write "控制1"(TRUE ("控制1")) -> ()
                n2242 = global write "EV05全局变量1.vi" "流控帧 2"(TRUE ("流控帧 2")) -> ()
                n2243 = local write "写?"(FALSE ("写?")) -> ()
                n2244 = local write "消除"(TRUE ("消除")) -> ()
              }
              frame #2 {
                n2245 = flat-sequence {
                  tunnel: [w2732] -> w2731
                  tunnel: w2731 -> [w2739]
                  frame #0 {
                    n2246 = while {
                      tunnel: [w2733] -> w2732
                      i -> [w2737]
                      stop <- w2734 stop-if-true
                      n2247 = local read "继电器超时处理"() -> (w2733:bool)
                      n2248 = Greater Or Equal?(x=w2737, y=20) -> (x >= y?=w2735:bool)
                      n2249 = Wait Until Next ms Multiple(millisecond multiple=u32 100 ("毫秒倍数")) -> ()  [unwired: 1 out]
                      n2250 = Or(x=w2733, y=w2735) -> (x .or. y?=w2734:bool)
                    }
                  }
                  frame #1 {
                    n2251 = case shown="假" w2739 {
                      frame False {
                        n2252 = local read "充电继电器"() -> (w2740:bool)
                        n2253 = Not(x=w2740) -> (.not. x?=w2741:bool)
                        n2254 = local write "充电继电器"(w2741) -> ()
                        n2255 = One Button Dialog(message="继电器处理超时" ("消息"), button name ("OK")="是" ("按钮名称（“确定”）")) -> ()  [unwired: 1 out]
                      }
                      frame True {
                      }
                    }
                  }
                }
              }
            }
          }
          event "风机继电器": Value Change {
            n2256 = event-data() -> ("NewVal"=w2744:bool)  [unwired: 6 out]
            n2257 = stacked-sequence {
              tunnel: w2744 -> [_ w2757 _]
              frame #0 {
                w2748 = FALSE ("继电器超时处理")
                n2258 = local write "继电器超时处理"(w2748) -> ()
                n2259 = local write "正级继电器 6"(w2748) -> ()
                n2260 = global write "EV05全局变量1.vi" "流控帧"(FALSE ("流控帧")) -> ()
                n2261 = local write "主从选择"(enum32{"主板", "从板"}."主板" ("主从选择")) -> ()
              }
              frame #1 {
                n2262 = case shown="真" w2757 {
                  selector: w2757 -> [w2771 w2791]
                  tunnel: [w2770 w2790] -> w2756
                  tunnel: [w2759 w2779] -> w2751
                  frame True {
                    w2767 = 256.0 ("y")
                    w2759 = u32 1 ("命令序号")
                    w2770 = u8 192 ("命令")
                    n2263 = local read "动作保持时间"() -> (w2768:dbl)
                    n2264 = Quotient & Remainder(x=w2768, y=w2767) -> (x-y*floor(x/y)=w2760:dbl, floor(x/y)=w2764:dbl)
                    n2265 = Quotient & Remainder(x=w2764, y=w2767) -> (x-y*floor(x/y)=w2761:dbl, floor(x/y)=w2765:dbl)
                    n2266 = Quotient & Remainder(x=w2765, y=w2767) -> (x-y*floor(x/y)=w2762:dbl, floor(x/y)=w2766:dbl)
                    n2267 = Boolean To (0,1)(Boolean=w2771) -> (0, 1=w2769:i16)
                    n2268 = local read "设备索引号"() -> (w2776:u16)
                    n2269 = local read "CAN卡类型"() -> (w2777:u32)
                    n2270 = Quotient & Remainder(x=w2766, y=w2767) -> (x-y*floor(x/y)=w2763:dbl)  [unwired: 1 out]
                    n2271 = local read "CAN端口"() -> (w2775:u16)
                    n2272 = Build Array(i16 6 ("元素"), w2769, w2763, w2762, w2761, w2760, 0.0 ("元素")) -> (w2773:dbl[])
                    n2273 = call "多帧发送机制(EV05).vi"("can卡类型"=w2777, "设备索引号"=w2776, "CAN端口"=w2775, "命令"=w2770, "板号"=u8 0, "命令序号"=w2759, "输入数据"=w2773) -> ()  [unwired: 2 in, 11 out]
                  }
                  frame False {
                    w2787 = 256.0 ("y")
                    w2779 = u32 1 ("命令序号")
                    w2790 = u8 192 ("命令")
                    n2274 = local read "动作保持时间"() -> (w2788:dbl)
                    n2275 = Quotient & Remainder(x=w2788, y=w2787) -> (x-y*floor(x/y)=w2780:dbl, floor(x/y)=w2784:dbl)
                    n2276 = Quotient & Remainder(x=w2784, y=w2787) -> (x-y*floor(x/y)=w2781:dbl, floor(x/y)=w2785:dbl)
                    n2277 = Quotient & Remainder(x=w2785, y=w2787) -> (x-y*floor(x/y)=w2782:dbl, floor(x/y)=w2786:dbl)
                    n2278 = Boolean To (0,1)(Boolean=w2791) -> (0, 1=w2789:i16)
                    n2279 = local read "设备索引号"() -> (w2796:u16)
                    n2280 = local read "CAN卡类型"() -> (w2797:u32)
                    n2281 = Quotient & Remainder(x=w2786, y=w2787) -> (x-y*floor(x/y)=w2783:dbl)  [unwired: 1 out]
                    n2282 = local read "CAN端口"() -> (w2795:u16)
                    n2283 = Build Array(i16 6 ("元素"), w2789, w2783, w2782, w2781, w2780, 0.0 ("元素")) -> (w2793:dbl[])
                    n2284 = call "多帧发送机制(EV05).vi"("can卡类型"=w2797, "设备索引号"=w2796, "CAN端口"=w2795, "命令"=w2790, "板号"=u8 0, "命令序号"=w2779, "输入数据"=w2793) -> ()  [unwired: 2 in, 11 out]
                  }
                }
                n2285 = local write "命令序号"(w2751) -> ()
                n2286 = local write "命令"(w2756) -> ()
                n2287 = local write "清BUFF"(FALSE ("清BUFF")) -> ()
                n2288 = local write "控制1"(TRUE ("控制1")) -> ()
                n2289 = global write "EV05全局变量1.vi" "流控帧 2"(TRUE ("流控帧 2")) -> ()
                n2290 = local write "写?"(FALSE ("写?")) -> ()
                n2291 = local write "消除"(TRUE ("消除")) -> ()
              }
              frame #2 {
                n2292 = flat-sequence {
                  tunnel: [w2799] -> w2798
                  tunnel: w2798 -> [w2806]
                  frame #0 {
                    n2293 = while {
                      tunnel: [w2800] -> w2799
                      i -> [w2804]
                      stop <- w2801 stop-if-true
                      n2294 = local read "继电器超时处理"() -> (w2800:bool)
                      n2295 = Greater Or Equal?(x=w2804, y=20) -> (x >= y?=w2802:bool)
                      n2296 = Wait Until Next ms Multiple(millisecond multiple=u32 100 ("毫秒倍数")) -> ()  [unwired: 1 out]
                      n2297 = Or(x=w2800, y=w2802) -> (x .or. y?=w2801:bool)
                    }
                  }
                  frame #1 {
                    n2298 = case shown="假" w2806 {
                      frame False {
                        n2299 = local read "风机继电器"() -> (w2807:bool)
                        n2300 = Not(x=w2807) -> (.not. x?=w2808:bool)
                        n2301 = local write "风机继电器"(w2808) -> ()
                        n2302 = One Button Dialog(message="继电器处理超时" ("消息"), button name ("OK")="是" ("按钮名称（“确定”）")) -> ()  [unwired: 1 out]
                      }
                      frame True {
                      }
                    }
                  }
                }
              }
            }
          }
          event "加热继电器(从)": Value Change {
            n2303 = event-data() -> ("NewVal"=w2811:bool)  [unwired: 6 out]
            n2304 = stacked-sequence {
              tunnel: w2811 -> [_ w2825 _]
              frame #0 {
                w2815 = FALSE ("继电器超时处理")
                n2305 = local write "正级继电器 7"(w2815) -> ()
                n2306 = local write "继电器超时处理"(w2815) -> ()
                n2307 = global write "EV05全局变量1.vi" "流控帧"(FALSE ("流控帧")) -> ()
                n2308 = local write "主从选择"(enum32{"主板", "从板"}."从板" ("主从选择")) -> ()
              }
              frame #1 {
                n2309 = case shown="真" w2825 {
                  selector: w2825 -> [w2840 w2860]
                  tunnel: [w2839 w2859] -> w2824
                  tunnel: [w2838 w2858] -> w2818
                  tunnel: [w2827 w2847] -> w2819
                  frame True {
                    w2835 = 256.0 ("y")
                    w2827 = u32 1 ("命令序号")
                    w2839 = u8 192 ("命令")
                    n2310 = local read "动作保持时间"() -> (w2836:dbl)
                    n2311 = Quotient & Remainder(x=w2836, y=w2835) -> (x-y*floor(x/y)=w2828:dbl, floor(x/y)=w2832:dbl)
                    n2312 = Quotient & Remainder(x=w2832, y=w2835) -> (x-y*floor(x/y)=w2829:dbl, floor(x/y)=w2833:dbl)
                    n2313 = Quotient & Remainder(x=w2833, y=w2835) -> (x-y*floor(x/y)=w2830:dbl, floor(x/y)=w2834:dbl)
                    n2314 = Quotient & Remainder(x=w2834, y=w2835) -> (x-y*floor(x/y)=w2831:dbl)  [unwired: 1 out]
                    n2315 = Boolean To (0,1)(Boolean=w2840) -> (0, 1=w2837:i16)
                    n2316 = local read "设备索引号"() -> (w2844:u16)
                    n2317 = local read "CAN卡类型"() -> (w2845:u32)
                    n2318 = local read "从板板号"() -> (w2838:u8)
                    n2319 = local read "CAN端口"() -> (w2843:u16)
                    n2320 = Build Array(i16 7 ("元素"), w2837, w2831, w2830, w2829, w2828, 0.0 ("元素")) -> (w2842:dbl[])
                    n2321 = call "多帧发送机制(EV05).vi"("can卡类型"=w2845, "设备索引号"=w2844, "CAN端口"=w2843, "命令"=w2839, "板号"=w2838, "命令序号"=w2827, "输入数据"=w2842) -> ()  [unwired: 2 in, 11 out]
                  }
                  frame False {
                    w2855 = 256.0 ("y")
                    w2847 = u32 1 ("命令序号")
                    w2859 = u8 192 ("命令")
                    n2322 = local read "动作保持时间"() -> (w2856:dbl)
                    n2323 = Quotient & Remainder(x=w2856, y=w2855) -> (x-y*floor(x/y)=w2848:dbl, floor(x/y)=w2852:dbl)
                    n2324 = Quotient & Remainder(x=w2852, y=w2855) -> (x-y*floor(x/y)=w2849:dbl, floor(x/y)=w2853:dbl)
                    n2325 = Quotient & Remainder(x=w2853, y=w2855) -> (x-y*floor(x/y)=w2850:dbl, floor(x/y)=w2854:dbl)
                    n2326 = Quotient & Remainder(x=w2854, y=w2855) -> (x-y*floor(x/y)=w2851:dbl)  [unwired: 1 out]
                    n2327 = Boolean To (0,1)(Boolean=w2860) -> (0, 1=w2857:i16)
                    n2328 = local read "设备索引号"() -> (w2864:u16)
                    n2329 = local read "CAN卡类型"() -> (w2865:u32)
                    n2330 = local read "从板板号"() -> (w2858:u8)
                    n2331 = local read "CAN端口"() -> (w2863:u16)
                    n2332 = Build Array(i16 7 ("元素"), w2857, w2851, w2850, w2849, w2848, 0.0 ("元素")) -> (w2862:dbl[])
                    n2333 = call "多帧发送机制(EV05).vi"("can卡类型"=w2865, "设备索引号"=w2864, "CAN端口"=w2863, "命令"=w2859, "板号"=w2858, "命令序号"=w2847, "输入数据"=w2862) -> ()  [unwired: 2 in, 11 out]
                  }
                }
                n2334 = local write "从板板号"(w2818) -> ()
                n2335 = local write "命令序号"(w2819) -> ()
                n2336 = local write "命令"(w2824) -> ()
                n2337 = local write "清BUFF"(FALSE ("清BUFF")) -> ()
                n2338 = local write "写?"(FALSE ("写?")) -> ()
                n2339 = local write "控制1"(TRUE ("控制1")) -> ()
                n2340 = global write "EV05全局变量1.vi" "流控帧 2"(TRUE ("流控帧 2")) -> ()
                n2341 = local write "消除"(TRUE ("消除")) -> ()
              }
              frame #2 {
                n2342 = flat-sequence {
                  tunnel: [w2867] -> w2866
                  tunnel: w2866 -> [w2874]
                  frame #0 {
                    n2343 = while {
                      tunnel: [w2868] -> w2867
                      i -> [w2872]
                      stop <- w2869 stop-if-true
                      n2344 = local read "继电器超时处理"() -> (w2868:bool)
                      n2345 = Greater Or Equal?(x=w2872, y=20) -> (x >= y?=w2870:bool)
                      n2346 = Wait Until Next ms Multiple(millisecond multiple=u32 100 ("毫秒倍数")) -> ()  [unwired: 1 out]
                      n2347 = Or(x=w2868, y=w2870) -> (x .or. y?=w2869:bool)
                    }
                  }
                  frame #1 {
                    n2348 = case shown="假" w2874 {
                      frame False {
                        n2349 = local read "加热继电器(从)"() -> (w2876:bool)
                        n2350 = Not(x=w2876) -> (.not. x?=w2875:bool)
                        n2351 = local write "加热继电器(从)"(w2875) -> ()
                        n2352 = One Button Dialog(message="继电器处理超时" ("消息"), button name ("OK")="是" ("按钮名称（“确定”）")) -> ()  [unwired: 1 out]
                      }
                      frame True {
                      }
                    }
                  }
                }
              }
            }
          }
          event "风机继电器(从)": Value Change {
            n2353 = event-data() -> ("NewVal"=w2879:bool)  [unwired: 6 out]
            n2354 = stacked-sequence {
              tunnel: w2879 -> [_ w2893 _]
              frame #0 {
                w2883 = FALSE ("继电器超时处理")
                n2355 = local write "继电器超时处理"(w2883) -> ()
                n2356 = local write "正级继电器 8"(w2883) -> ()
                n2357 = global write "EV05全局变量1.vi" "流控帧"(FALSE ("流控帧")) -> ()
                n2358 = local write "主从选择"(enum32{"主板", "从板"}."从板" ("主从选择")) -> ()
              }
              frame #1 {
                n2359 = case shown="假" w2893 {
                  selector: w2893 -> [w2908 w2928]
                  tunnel: [w2907 w2927] -> w2892
                  tunnel: [w2906 w2926] -> w2886
                  tunnel: [w2895 w2915] -> w2887
                  frame False {
                    w2903 = 256.0 ("y")
                    w2895 = u32 1 ("命令序号")
                    w2907 = u8 192 ("命令")
                    n2360 = local read "动作保持时间"() -> (w2904:dbl)
                    n2361 = Quotient & Remainder(x=w2904, y=w2903) -> (x-y*floor(x/y)=w2896:dbl, floor(x/y)=w2900:dbl)
                    n2362 = Quotient & Remainder(x=w2900, y=w2903) -> (x-y*floor(x/y)=w2897:dbl, floor(x/y)=w2901:dbl)
                    n2363 = Quotient & Remainder(x=w2901, y=w2903) -> (x-y*floor(x/y)=w2898:dbl, floor(x/y)=w2902:dbl)
                    n2364 = Quotient & Remainder(x=w2902, y=w2903) -> (x-y*floor(x/y)=w2899:dbl)  [unwired: 1 out]
                    n2365 = local read "设备索引号"() -> (w2912:u16)
                    n2366 = local read "CAN卡类型"() -> (w2913:u32)
                    n2367 = local read "从板板号"() -> (w2906:u8)
                    n2368 = Boolean To (0,1)(Boolean=w2908) -> (0, 1=w2905:i16)
                    n2369 = local read "CAN端口"() -> (w2911:u16)
                    n2370 = Build Array(i16 8 ("元素"), w2905, w2899, w2898, w2897, w2896, 0.0 ("元素")) -> (w2910:dbl[])
                    n2371 = call "多帧发送机制(EV05).vi"("can卡类型"=w2913, "设备索引号"=w2912, "CAN端口"=w2911, "命令"=w2907, "板号"=w2906, "命令序号"=w2895, "输入数据"=w2910) -> ()  [unwired: 2 in, 11 out]
                  }
                  frame True {
                    w2923 = 256.0 ("y")
                    w2915 = u32 1 ("命令序号")
                    w2927 = u8 192 ("命令")
                    n2372 = local read "动作保持时间"() -> (w2924:dbl)
                    n2373 = Quotient & Remainder(x=w2924, y=w2923) -> (x-y*floor(x/y)=w2916:dbl, floor(x/y)=w2920:dbl)
                    n2374 = Quotient & Remainder(x=w2920, y=w2923) -> (x-y*floor(x/y)=w2917:dbl, floor(x/y)=w2921:dbl)
                    n2375 = Quotient & Remainder(x=w2921, y=w2923) -> (x-y*floor(x/y)=w2918:dbl, floor(x/y)=w2922:dbl)
                    n2376 = Quotient & Remainder(x=w2922, y=w2923) -> (x-y*floor(x/y)=w2919:dbl)  [unwired: 1 out]
                    n2377 = local read "设备索引号"() -> (w2932:u16)
                    n2378 = local read "CAN卡类型"() -> (w2933:u32)
                    n2379 = local read "从板板号"() -> (w2926:u8)
                    n2380 = Boolean To (0,1)(Boolean=w2928) -> (0, 1=w2925:i16)
                    n2381 = local read "CAN端口"() -> (w2931:u16)
                    n2382 = Build Array(i16 8 ("元素"), w2925, w2919, w2918, w2917, w2916, 0.0 ("元素")) -> (w2930:dbl[])
                    n2383 = call "多帧发送机制(EV05).vi"("can卡类型"=w2933, "设备索引号"=w2932, "CAN端口"=w2931, "命令"=w2927, "板号"=w2926, "命令序号"=w2915, "输入数据"=w2930) -> ()  [unwired: 2 in, 11 out]
                  }
                }
                n2384 = local write "从板板号"(w2886) -> ()
                n2385 = local write "清BUFF"(FALSE ("清BUFF")) -> ()
                n2386 = local write "命令序号"(w2887) -> ()
                n2387 = local write "命令"(w2892) -> ()
                n2388 = local write "控制1"(TRUE ("控制1")) -> ()
                n2389 = local write "写?"(FALSE ("写?")) -> ()
                n2390 = local write "消除"(TRUE ("消除")) -> ()
                n2391 = global write "EV05全局变量1.vi" "流控帧 2"(TRUE ("流控帧 2")) -> ()
              }
              frame #2 {
                n2392 = flat-sequence {
                  tunnel: [w2935] -> w2934
                  tunnel: w2934 -> [w2942]
                  frame #0 {
                    n2393 = while {
                      tunnel: [w2936] -> w2935
                      i -> [w2940]
                      stop <- w2937 stop-if-true
                      n2394 = local read "继电器超时处理"() -> (w2936:bool)
                      n2395 = Greater Or Equal?(x=w2940, y=20) -> (x >= y?=w2938:bool)
                      n2396 = Wait Until Next ms Multiple(millisecond multiple=u32 100 ("毫秒倍数")) -> ()  [unwired: 1 out]
                      n2397 = Or(x=w2936, y=w2938) -> (x .or. y?=w2937:bool)
                    }
                  }
                  frame #1 {
                    n2398 = case shown="假" w2942 {
                      frame False {
                        n2399 = local read "风机继电器(从)"() -> (w2944:bool)
                        n2400 = Not(x=w2944) -> (.not. x?=w2943:bool)
